vi "Configure Multi Eval Meas Limit EVM.vi"(4 "Peak (60.0)":dbl=60.0, 5 "Peak Enabled (Off)":i32(ring) items=["Off", "On", "Value"], 6 "RMS (30.0)":dbl=30.0, 7 "RMS Enabled (Value)":i32(ring)=2 items=["Off", "On", "Value"], 8 "error in (no error)":errorcluster, 9 "Modulation (Pi/2-BPSK)":i32(ring) items=["Pi/2-BPSK"=0, "Pi/2-BPSK With Shaping"=5, "QPSK"=1, "16-QAM"=2, "64-QAM"=3, "256-QAM"=4], 10 "Instance (1)":T1=1, 11 "VISA resource name":refnum<visa-resource-name>) -> (0 "error out":errorcluster, 3 "VISA resource name out":refnum<visa-resource-name>)   [LabVIEW 2020, in "Rohde&Schwarz CMWXP NR FR1 Measurement.lvlib"]
doc: "Defines upper limits for the RMS and peak values of the error vector magnitude (EVM) for selected modulation scheme.\n\nAttributes:\nRSCMWXPNRFR1M_ATTR_MULTI_EVAL_MEAS_LIMIT_PI_2_EVM\nRSCMWXPNRFR1M_ATTR_MULTI_EVAL_MEAS_LIMIT_BPSK_SHAPING_EVM\nRSCMWXPNRFR1M_ATTR_MULTI_EVAL_MEAS_LIMIT_QPSK_EVM\nRSCMWXPNRFR1M_ATTR_MULTI_EVAL_MEAS_LIMIT_QAM_EVM\n\nRemote-control commands:\nCONFigure:NRSub:MEAS<i>:MEValuation:LIMit:PHBPsk:EVMagnitude\nCONFigure:NRSub:MEAS<i>:MEValuation:LIMit:BPWShaping:EVMagnitude\nCONFigure:NRSub:MEAS<i>:MEValuation:LIMit:QPSK:EVMagnitude\nCONFigure:NRSub:MEAS<i>:MEValuation:LIMit:QAM<order>:EVMagnitude"
uses:
  <instrlib>/Rohde&Schwarz CMWXP NR FR1 Measurement/Rohde&Schwarz CMWXP NR FR1 Measurement.lvlib
  <instrlib>/Rohde&Schwarz CMWXP NR FR1 Measurement/Private/_Instance.ctl
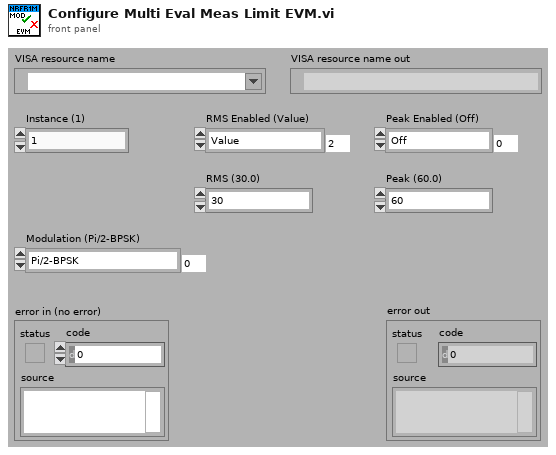
[diagram p1: front panel]
types:
  T1 = typedef "Rohde&Schwarz CMWXP NR FR1 Measurement.lvlib/_Instance.ctl" = i32
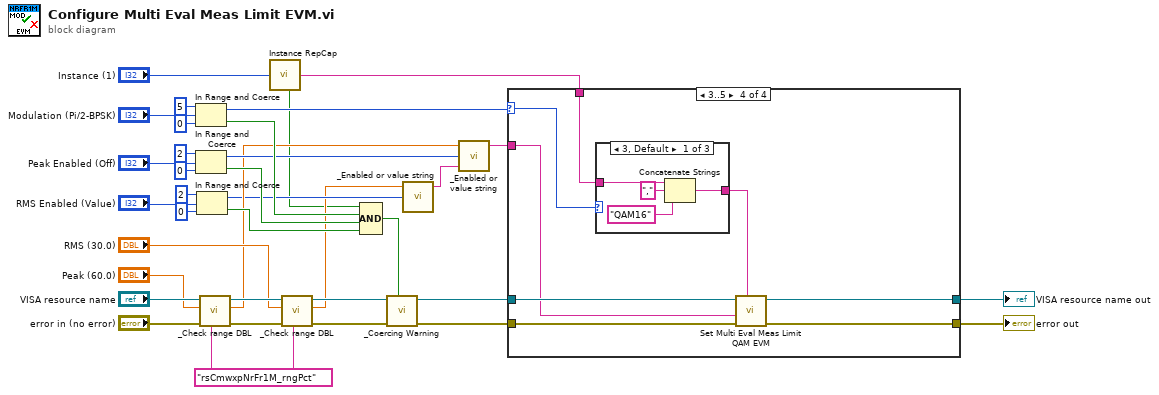
[diagram p0: block diagram]
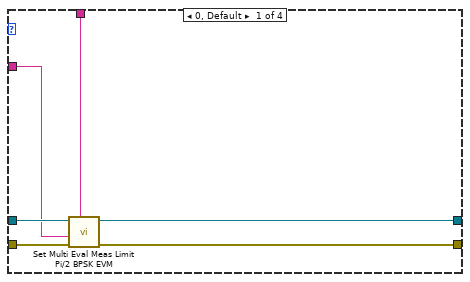
[diagram p2: hidden frame]
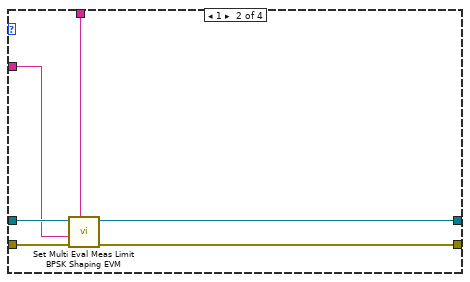
[diagram p3: hidden frame]
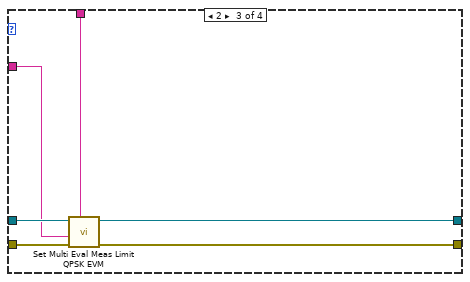
[diagram p4: hidden frame]
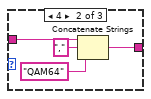
[diagram p5: hidden frame]
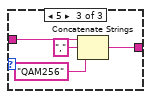
[diagram p6: hidden frame]
diagram:
  w24 = "rsCmwxpNrFr1M_rngPct" ("Range Table Identifier")
  n1 = In Range and Coerce(upper limit=5, x="Modulation (Pi/2-BPSK)", lower limit=0) -> (coerced(x)=w4:i32, In Range?=w17:bool)
  n2 = In Range and Coerce(upper limit=2, x="Peak Enabled (Off)", lower limit=0) -> (coerced(x)=w8:i32, In Range?=w16:bool)
  n3 = In Range and Coerce(upper limit=2, x="RMS Enabled (Value)", lower limit=0) -> (coerced(x)=w6:i32, In Range?=w15:bool)
  n4 = call <instrlib>:"_Check range DBL.vi"("Range Table Identifier"=w24, "error in (no error)"="error in (no error)", "DBL Value In"="Peak (60.0)", "VISA resource name"="VISA resource name") -> ("error out"=w27:errorcluster, "DBL Value Out"=w7:dbl, "VISA resource name out"=w26:refnum<visa-resource-name>)  [unwired: 5 in]
  n5 = call <instrlib>:"Instance RepCap.vi"("Instance In"="Instance (1)") -> ("In Range?"=w1:bool, "RepCap Identifier Out"=w9:string)  [unwired: 1 in]
  n6 = call <instrlib>:"_Check range DBL.vi"("Range Table Identifier"=w24, "error in (no error)"=w27, "DBL Value In"="RMS (30.0)", "VISA resource name"=w26) -> ("error out"=w19:errorcluster, "DBL Value Out"=w5:dbl, "VISA resource name out"=w18:refnum<visa-resource-name>)  [unwired: 5 in]
  n7 = Compound Arithmetic op=AND(w1, w17, w16, w15) -> (w14:bool)
  n8 = call <instrlib>:"_Coercing Warning.vi"("In Range?"=w14, "error in (no error)"=w19, "VISA resource name"=w18) -> ("error out"=w13:errorcluster, "VISA resource name out"=w10:refnum<visa-resource-name>)  [unwired: 7 in]
  n9 = call <instrlib>:"_Enabled or value string.vi"("Enabled or Value"=w6, "Value"=w5) -> ("Resulting String"=w2:string)  [unwired: 3 in]
  n10 = call <instrlib>:"_Enabled or value string.vi"("Initial String"=w2, "Enabled or Value"=w8, "Value"=w7) -> ("Resulting String"=w3:string)  [unwired: 2 in]
  n11 = case shown="3..5" w4 {
    selector: w4 -> [_ _ _ w57]
    tunnel: w13 -> [w42 w48 w54 w62]
    tunnel: [w41 w47 w53 w61] -> w12
    tunnel: [w40 w46 w52 w60] -> w11
    tunnel: w10 -> [w39 w45 w51 w59]
    tunnel: w9 -> [w38 w44 w50 w56]
    tunnel: w3 -> [w37 w43 w49 w58]
    frame 0, Default {
      n12 = call "Set Multi Eval Meas Limit Pi/2 BPSK EVM"("Repeated Capabilities"=w38, "error in (no error)"=w42, "Multi Eval Meas Limit Pi/2 BPSK EVM ()"=w37, "instrument handle"=w39) -> ("error out"=w41:errorcluster, "instrument handle out"=w40:refnum<visa-resource-name>)  [unwired: 6 in]
    }
    frame 1 {
      n13 = call "Set Multi Eval Meas Limit BPSK Shaping EVM"("Repeated Capabilities"=w44, "error in (no error)"=w48, "Multi Eval Meas Limit BPSK Shaping EVM ()"=w43, "instrument handle"=w45) -> ("error out"=w47:errorcluster, "instrument handle out"=w46:refnum<visa-resource-name>)  [unwired: 6 in]
    }
    frame 2 {
      n14 = call "Set Multi Eval Meas Limit QPSK EVM"("Repeated Capabilities"=w50, "error in (no error)"=w54, "Multi Eval Meas Limit QPSK EVM ()"=w49, "instrument handle"=w51) -> ("error out"=w53:errorcluster, "instrument handle out"=w52:refnum<visa-resource-name>)  [unwired: 6 in]
    }
    frame 3..5 {
      n15 = case shown="3, Default" w57 {
        tunnel: w56 -> [w66 w70 w74]
        tunnel: [w65 w69 w73] -> w55
        frame 3, Default {
          n16 = Concatenate Strings(w66, "," ("string"), "QAM16" ("string")) -> (w65:string)
        }
        frame 4 {
          n17 = Concatenate Strings(w70, "," ("string"), "QAM64" ("string")) -> (w69:string)
        }
        frame 5 {
          n18 = Concatenate Strings(w74, "," ("string"), "QAM256" ("string")) -> (w73:string)
        }
      }
      n19 = call "Set Multi Eval Meas Limit QAM EVM"("Repeated Capabilities"=w55, "error in (no error)"=w62, "Multi Eval Meas Limit QAM EVM ()"=w58, "instrument handle"=w59) -> ("error out"=w61:errorcluster, "instrument handle out"=w60:refnum<visa-resource-name>)  [unwired: 6 in]
    }
  }
  "error out" <- w12
  "VISA resource name out" <- w11
